vi "take_element_type.vi"(10 "BSONbytes":u8[](array[numeric])) -> (2 "restOfBytes":u8[](array[numeric]), 3 "dataType":T1)   [LabVIEW 2015, in "BSON_convertors_Library.lvlib"]
uses:
  BSON_convertors_Library.lvlib
  typedefs/dataType.ctl
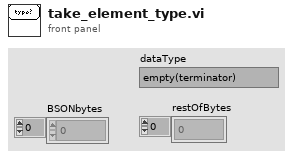
[diagram p1: front panel]
types:
  T1 = typedef "BSON_convertors_Library.lvlib/dataType.ctl" = enum8{"empty(terminator)", "double", "string", "document", "array", "binary", "Deprecated(Undefined)", "ObjectId", "boolean", "UTC datetime", "Null value", "cstring", "Deprecated(DBPointer)", "JavaScript", "Deprecated(Symbol)", "code_w_s", "int32", "uint64", "int64", "ext (decimal128)", "Min key", "Max key"}
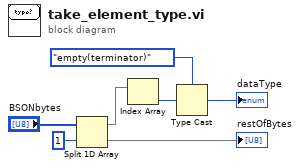
[diagram p0: block diagram]
diagram:
  n1 = Split 1D Array(array="BSONbytes", index=1) -> (first subarray=w5:u8[], second subarray=→"restOfBytes":u8[])
  n2 = Index Array(array=w5) -> (element=w6:u8)  [unwired: 1 in]
  n3 = Type Cast(type=dataType."empty(terminator)" ("dataType"), x=w6) -> (*(type *) &x=→"dataType":T1)
